vi "XY Sample Stage Mark Points Holder.vi"(0 "Index":i32, 2 "Actions":T1=enum."Read", 7 "(X, Y) Points":dbl[](array[numeric])) -> (4 "Marked Points":cluster{dbl[], dbl[]})   [LabVIEW 2020]
uses:
  XY Sample Stage Controls/XY Sample Stage History Actions.ctl
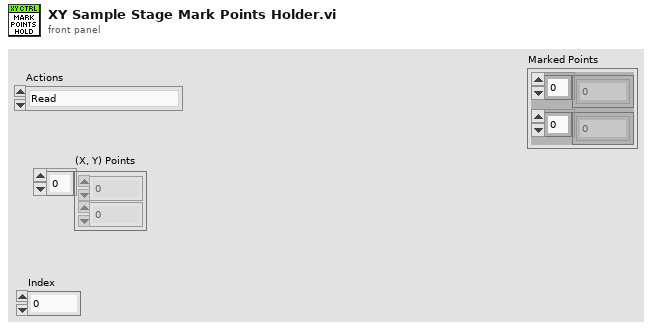
[diagram p1: front panel]
types:
  T1 = typedef "XY Sample Stage History Actions.ctl" = enum16{"Reset", "Write", "Read", "Set Zero", "Update", "Remove"}
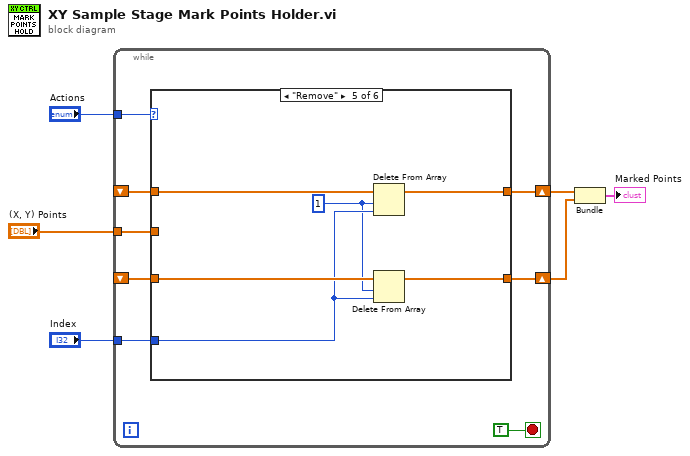
[diagram p0: block diagram]
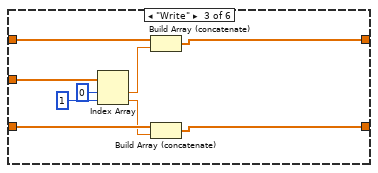
[diagram p4: hidden frame]
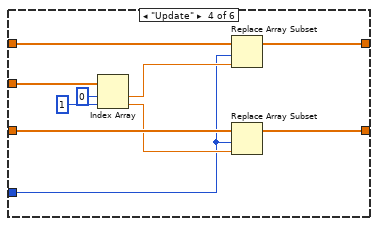
[diagram p5: hidden frame]
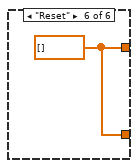
[diagram p6: hidden frame]
diagram:
  n1 = while {
    shift-right: [w12] -> w4
    shift-left: _ -> [w10]
    shift-right: [w11] -> w3
    shift-left: _ -> [w9]
    tunnel: "Actions" -> [w13]
    tunnel: "(X, Y) Points" -> [w8]
    tunnel: "Index" -> [w7]
    stop <- TRUE stop-if-true
    n2 = case shown="\"Remove\"" w13 {
      tunnel: [w16 w18 w21 w33 w42 w44] -> w12
      tunnel: [w15 w17 w20 w31 w40 w44] -> w11
      tunnel: w10 -> [w16 w18 w27 w34 w43 _]
      tunnel: w9 -> [w15 w17 w26 w32 w41 _]
      tunnel: w8 -> [_ _ w19 w35 _ _]
      tunnel: w7 -> [_ _ _ w28 w39 _]
      frame "Read", Default {
      }
      frame "Set Zero" {
      }
      frame "Write" {
        n3 = Index Array(array=w19, index #1=0 ("index"), index #2=1 ("index")) -> (element #1=w23:dbl, element #2=w22:dbl)
        n4 = Build Array (concatenate)(w27, w23) -> (w21:dbl[])
        n5 = Build Array (concatenate)(w26, w22) -> (w20:dbl[])
      }
      frame "Update" {
        n6 = Index Array(array=w35, index #1=0 ("index"), index #2=1 ("index")) -> (element #1=w30:dbl, element #2=w29:dbl)
        n7 = Replace Array Subset(array=w34, new element=w30, index=w28) -> (w33:dbl[])
        n8 = Replace Array Subset(array=w32, new element=w29, index=w28) -> (w31:dbl[])
      }
      frame "Remove" {
        w38 = 1 ("length")
        n9 = Delete From Array(array=w43, length=w38, index=w39) -> (array with subset deleted=w42:dbl[])  [unwired: 1 out]
        n10 = Delete From Array(array=w41, length=w38, index=w39) -> (array with subset deleted=w40:dbl[])  [unwired: 1 out]
      }
      frame "Reset" {
        w44 = dbl[] []
      }
    }
  }
  n11 = Bundle(w4, w3) -> (→"Marked Points":cluster{dbl[], dbl[]})  [unwired: 1 in]
